vi "PM5000_Power_Metering.vi"(8 "error in":errorcluster, 11 "Network Path":string="172.22.26.202") -> (0 "error out":errorcluster, 1 "Power_array":sgl[](array[numeric]), 2 "Power Meter Out":T1, 3 "Network Path out":string="192.168.169.1")   [LabVIEW 2018]
doc: "Lee la tabla de memoria RealTime_VIF_Power del equipo PowerMonitor 5000, ademas filtra y ordena las variables de interez de la tabla de memoria.\n\nLee las siguientes variables de la tabla RealTime_VIF_Power:\n\n*V1_V2_Volts\n*V2_V3_Volts\n*V3_V1_Volts\n*I1_Amps\n*I2_Amps\n*I3_Amps\n*Frequency_Hz\n*Total_kW\n*Total_kVAR\n*Total_kVA\n*Total_True_PF\n*Total_Disp_PF"
uses:
  <vilib>/ethernetip/ethernetip.llb/EthernetIP SLC500 Read Float.vi
  <vilib>/ethernetip/ethernetip.lvlib
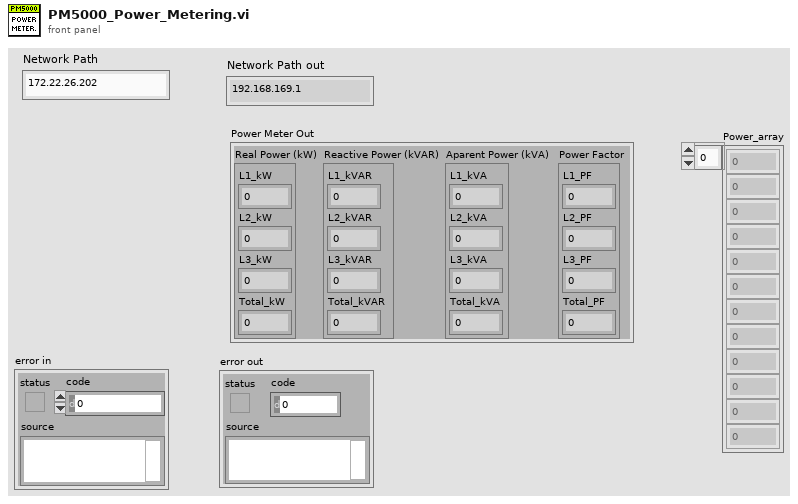
[diagram p1: front panel]
types:
  T1 = cluster{"Real Power (kW)":cluster{"L1_kW":sgl, "L2_kW":sgl, "L3_kW":sgl, "Total_kW":sgl}, "Reactive Power (kVAR)":cluster{"L1_kVAR":sgl, "L2_kVAR":sgl, "L3_kVAR":sgl, "Total_kVAR":sgl}, "Aparent Power (kVA)":cluster{"L1_kVA":sgl, "L2_kVA":sgl, "L3_kVA":sgl, "Total_kVA":sgl}, "Power Factor":cluster{"L1_PF":sgl, "L2_PF":sgl, "L3_PF":sgl, "Total_PF":sgl}}
  T2 = cluster{"Real Power (kW)":cluster{"L1_kW":sgl, "L2_kW":sgl, "L3_kW":sgl, "Total_kW":sgl}, "Reactive Power (kVAR)":cluster{"L1_kVAR":sgl, "L2_kVAR":sgl, "L3_kVAR":sgl, "Total_kVAR":sgl}, "Aparent Power (kVA)":cluster{"L1_kVA":sgl, "L2_kVA":sgl, "L3_kVA":sgl, "Total_kVA":sgl}, "Power Factor (%)":cluster{"L1_PF":sgl, "L2_PF":sgl, "L3_PF":sgl, "Total_PF":sgl}}
  T3 = cluster{"L1_PF":sgl, "L2_PF":sgl, "L3_PF":sgl, "Total_PF":sgl}
  T4 = cluster{"L1_kVA":sgl, "L2_kVA":sgl, "L3_kVA":sgl, "Total_kVA":sgl}
  T5 = cluster{"L1_kVAR":sgl, "L2_kVAR":sgl, "L3_kVAR":sgl, "Total_kVAR":sgl}
  T6 = cluster{"L1_kW":sgl, "L2_kW":sgl, "L3_kW":sgl, "Total_kW":sgl}
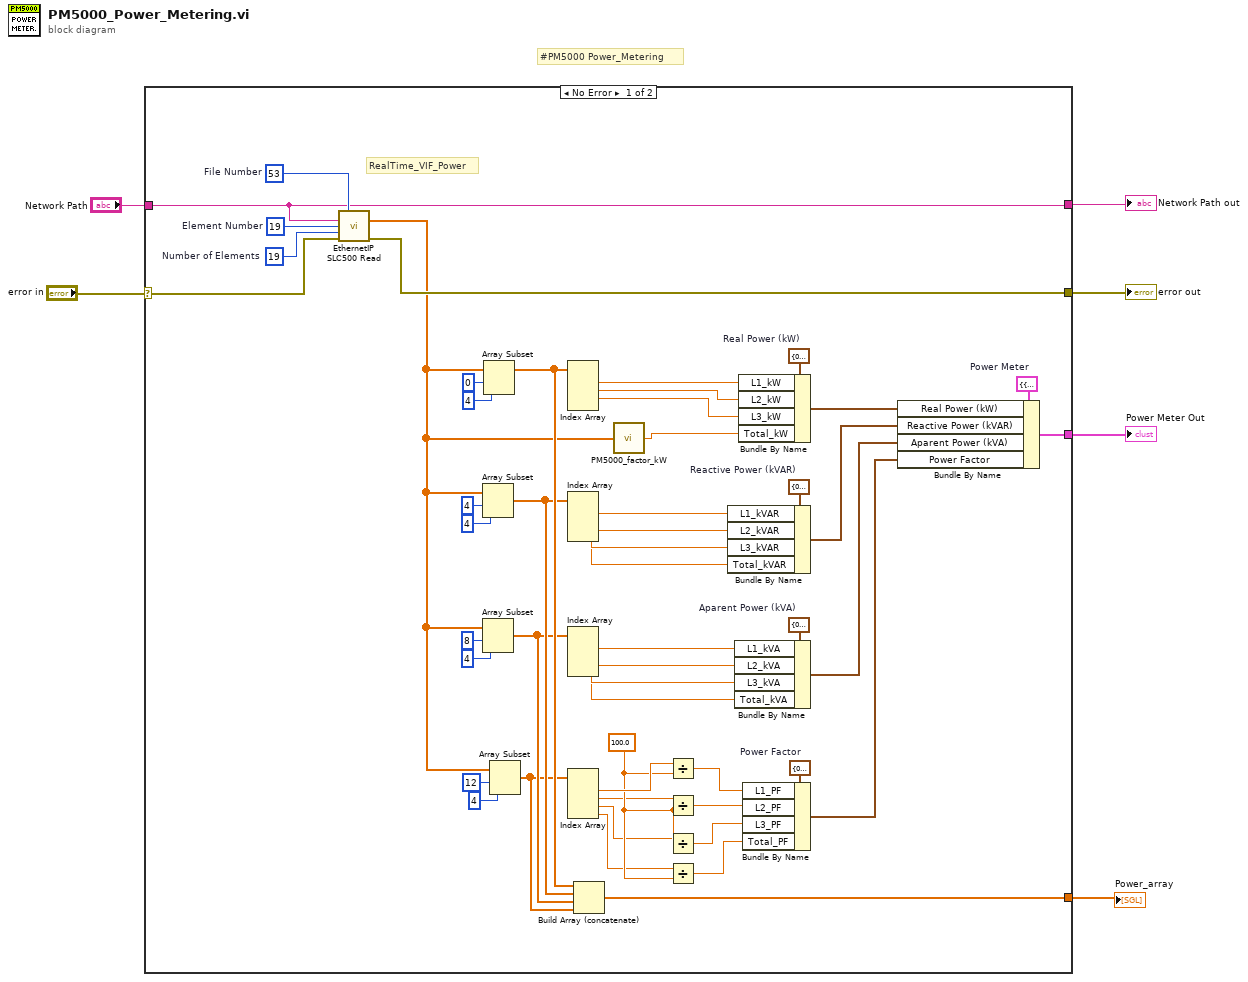
[diagram p0: block diagram]
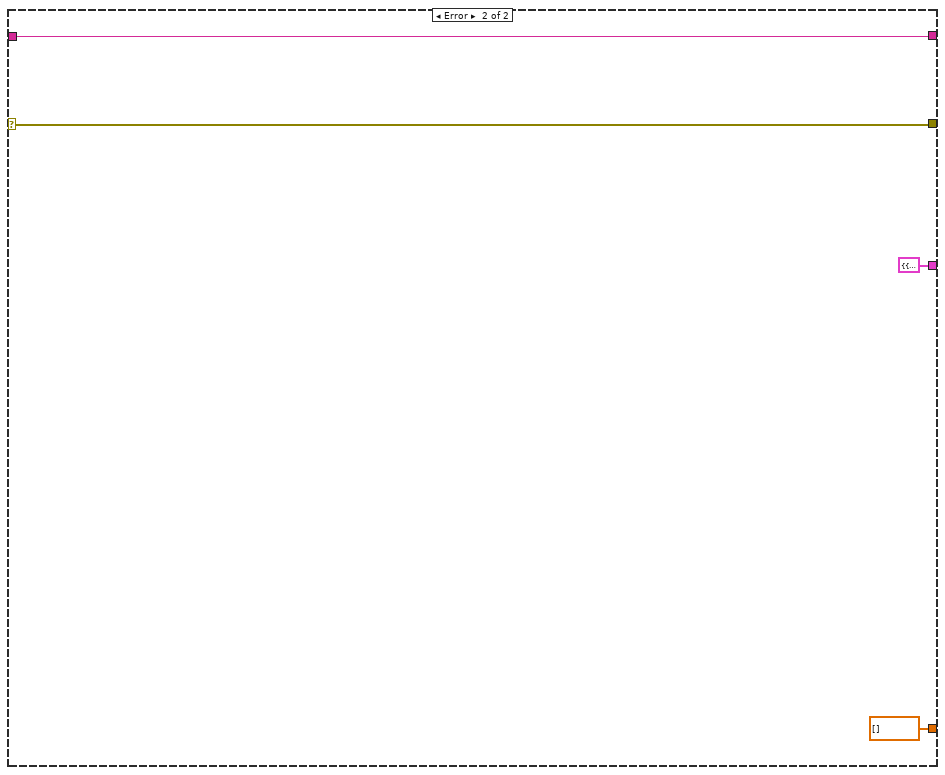
[diagram p2: hidden frame]
diagram:
  # "#PM5000 Power_Metering"
  n1 = case shown="No Error" "error in" {
    selector: "error in" -> [w24 w61]
    tunnel: [w57 w61] -> w6
    tunnel: [w19 w59] -> w5
    tunnel: [w25 T2 {"Real Power (kW)"={"L1_kW"=0.0, "L2_kW"=0.0, "L3_kW"=0.0, "Total_kW"=0.0}, "Reactive Power (kVAR)"={"L1_kVAR"=0.0, "L2_kVAR"=0.0, "L3_kVAR"=0.0, "Total_kVAR"=0.0}, "Aparent Power (kVA)"={"L1_kVA"=0.0, "L2_kVA"=0.0, "L3_kVA"=0.0, "Total_kVA"=0.0}, "Power Factor (%)"={"L1_PF"=0.0, "L2_PF"=0.0, "L3_PF"=0.0, "Total_PF"=0.0}} ("Power Meter")] -> w4
    tunnel: "Network Path" -> [w19 w59]
    tunnel: [w18 sgl[] []] -> w1
    frame No Error {
      w16 = sgl 100.0 ("y")
      w30 = T1 {"Real Power (kW)"={"L1_kW"=-0.009145112, "L2_kW"=-0.0037322815, "L3_kW"=-0.019452685, "Total_kW"=-0.03233008}, "Reactive Power (kVAR)"={"L1_kVAR"=-0.01587091, "L2_kVAR"=-0.0369946, "L3_kVAR"=-0.038295496, "Total_kVAR"=-0.091161005}, "Aparent Power (kVA)"={"L1_kVA"=0.018485848, "L2_kVA"=0.037469197, "L3_kVA"=0.04338286, "Total_kVA"=0.099337906}, "Power Factor"={"L1_PF"=49.470882, "L2_PF"=9.960934, "L3_PF"=44.839565, "Total_PF"=32.545567}}  # Power Meter
      w47 = T3 {"L1_PF"=0.0, "L2_PF"=0.0, "L3_PF"=0.0, "Total_PF"=0.0}  # Power Factor
      w48 = T4 {"L1_kVA"=0.0, "L2_kVA"=0.0, "L3_kVA"=0.0, "Total_kVA"=0.0}  # Aparent Power (kVA)
      w49 = T5 {"L1_kVAR"=0.0, "L2_kVAR"=0.0, "L3_kVAR"=0.0, "Total_kVAR"=0.0}  # Reactive Power (kVAR)
      w53 = T6 {"L1_kW"=0.0, "L2_kW"=0.0, "L3_kW"=0.0, "Total_kW"=0.0}  # Real Power (kW)
      w54 = u32 19  # Number of Elements
      w56 = u16 53  # File Number
      w55 = u16 19  # Element Number
      # "RealTime_VIF_Power"
      n2 = call-poly <vilib>:"EthernetIP SLC500 Read.vi"("File Number"=w56, "Network Path"=w19, "Element Number"=w55, "Number of Elements"=w54, "error in"=w24) -> ("Data"=w8:sgl[], "error out"=w57:errorcluster)  [unwired: 8 in, 1 out]
      n3 = Array Subset(array=w8, index=4, length=4) -> (w22:sgl[])
      n4 = Array Subset(array=w8, index=8, length=4) -> (w21:sgl[])
      n5 = Array Subset(array=w8, index=0, length=4) -> (w23:sgl[])
      n6 = Array Subset(array=w8, index=12, length=4) -> (w20:sgl[])
      n7 = Index Array(array=w23) -> (element #1=w52:sgl, element #2=w51:sgl, element #3=w50:sgl)  [unwired: 4 in, 1 out]
      n8 = Index Array(array=w22) -> (element #1=w38:sgl, element #2=w37:sgl, element #3=w36:sgl, element #4=w35:sgl)  [unwired: 4 in]
      n9 = Index Array(array=w21) -> (element #1=w34:sgl, element #2=w33:sgl, element #3=w32:sgl, element #4=w31:sgl)  [unwired: 4 in]
      n10 = Index Array(array=w20) -> (element #1=w17:sgl, element #2=w15:sgl, element #3=w14:sgl, element #4=w13:sgl)  [unwired: 4 in]
      n11 = Build Array (concatenate)(w23, w22, w21, w20) -> (w18:sgl[])
      n12 = call "PM5000_factor_kW.vi"("Data In"=w8) -> ("kW"=w7:sgl)
      n13 = Divide(x=w17, y=w16) -> (x/y=w12:sgl)
      n14 = Divide(x=w15, y=w16) -> (x/y=w11:sgl)
      n15 = Divide(x=w14, y=w16) -> (x/y=w10:sgl)
      n16 = Divide(x=w13, y=w16) -> (x/y=w9:sgl)
      n17 = Bundle By Name(cluster=w49, "L1_kVAR"=w38, "L2_kVAR"=w37, "L3_kVAR"=w36, "Total_kVAR"=w35) -> (w28:T5)
      n18 = Bundle By Name(cluster=w48, "L1_kVA"=w34, "L2_kVA"=w33, "L3_kVA"=w32, "Total_kVA"=w31) -> (w27:T4)
      n19 = Bundle By Name(cluster=w53, "L1_kW"=w52, "L2_kW"=w51, "L3_kW"=w50, "Total_kW"=w7) -> (w29:T6)
      n20 = Bundle By Name(cluster=w47, "L1_PF"=w12, "L2_PF"=w11, "L3_PF"=w10, "Total_PF"=w9) -> (w26:T3)
      n21 = Bundle By Name(cluster=w30, "Real Power (kW)"=w29, "Reactive Power (kVAR)"=w28, "Aparent Power (kVA)"=w27, "Power Factor"=w26) -> (w25:T1)
    }
    frame Error {
    }
  }
  "error out" <- w6
  "Network Path out" <- w5
  "Power Meter Out" <- w4
  "Power_array" <- w1
